vi "Control_PP_Blocks.vi"() -> (5 "Plug in titles":string[](array[string]), 7 "Plug in values":string[](array[string]))   [LabVIEW 2022 SP3]
uses:
  Globals/Meas_global.vi
  Post_Processing_specials/Block_Control_global.vi
panel:
  in  "No of Blocks to PP":i32=1 min=1
  in  "Start Block Number":i32=1 min=1
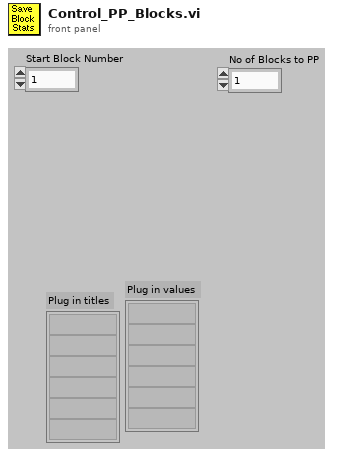
[diagram p1: front panel]
types:
  T1 = typedef "Post_Process.ctl" = enum16{"Take New Data", "Post Process Raw Data File"}
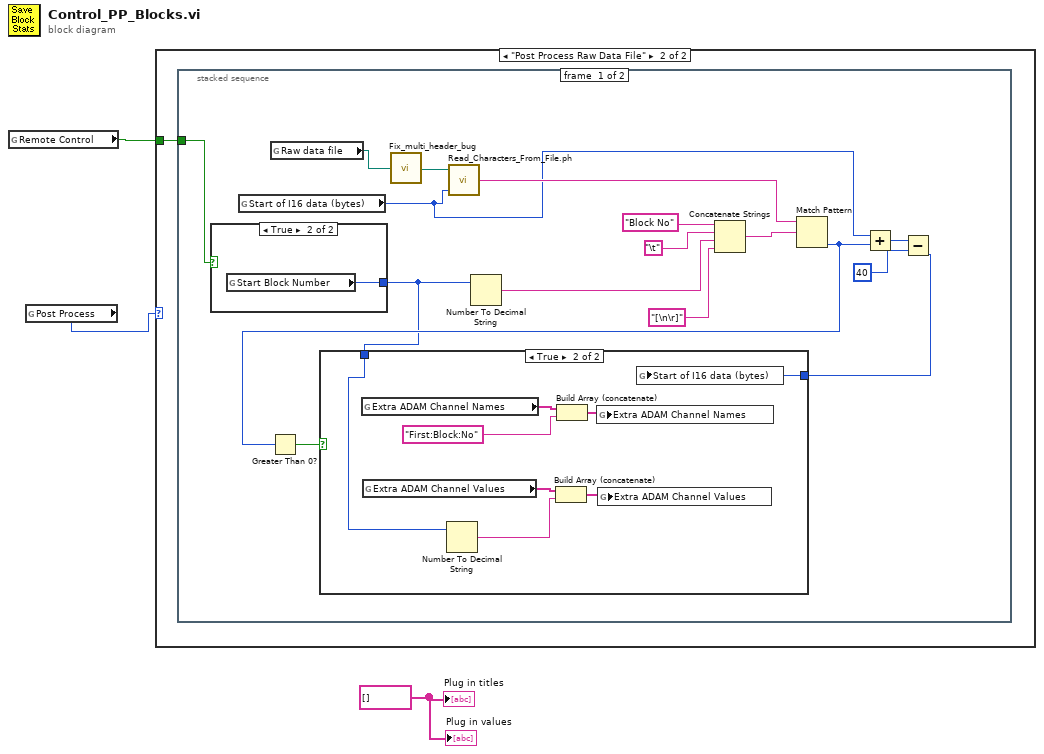
[diagram p0: block diagram]
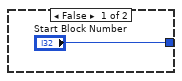
[diagram p3: hidden frame]
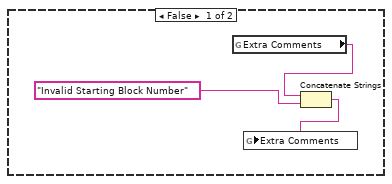
[diagram p4: hidden frame]
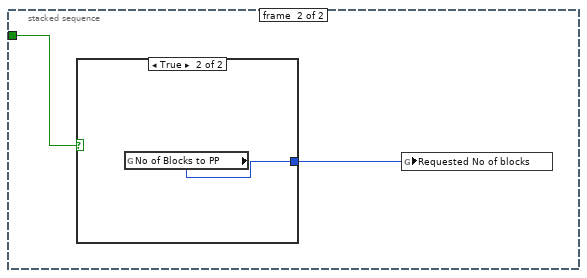
[diagram p5: hidden frame]
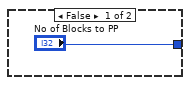
[diagram p6: hidden frame]
diagram:
  w2 = string[] [] ("Plug in titles")
  n1 = global read "Block_Control_global.vi" "Remote Control"() -> (w1:bool)
  n2 = global read "Meas_global.vi" "Post Process"() -> (w3:T1)
  n3 = case shown="\"Post Process Raw Data File\"" w3 {
    tunnel: w1 -> [_ w4]
    frame "Take New Data" {
    }
    frame "Post Process Raw Data File" {
      n4 = stacked-sequence {
        tunnel: w4 -> [w6 w34]
        frame #0 {
          n5 = case shown="True" w6 {
            tunnel: ["Start Block Number" w22] -> w5
            frame False {
            }
            frame True {
              n6 = global read "Block_Control_global.vi" "Start Block Number"() -> (w22:i32)
            }
          }
          n7 = global read "Meas_global.vi" "Start of I16 data (bytes)"() -> (w12:i64)
          n8 = global read "Meas_global.vi" "Raw data file"() -> (w20:path)
          n9 = call "Fix_multi_header_bug.vi"("Raw data File to Read"=w20) -> ("Raw data File to Read Out"=w19:path)
          n10 = call "Read_Characters_From_File.ph.vi"("file path (dialog if empty)"=w19, "start of read offset (chars.: 0)"=w12) -> ("character string"=w14:string)  [unwired: 4 in, 3 out]
          n11 = Number To Decimal String(number=w5) -> (decimal integer string=w16:string)  [unwired: 1 in]
          n12 = Concatenate Strings("Block No", "\t", w16, "[\n\r]") -> (w15:string)
          n13 = Match Pattern(string=w14, regular expression=w15) -> (offset past match=w9:i32)  [unwired: 1 in, 3 out]
          n14 = Greater Than 0?(x=w9) -> (x > 0?=w8:bool)
          n15 = Add(x=w12, y=w9) -> (x+y=w11:i64)
          n16 = Subtract(x=w11, y=40) -> (x-y=w7:i64)
          n17 = case shown="True" w8 {
            tunnel: w7 -> [_ w33]
            tunnel: w5 -> [_ w27]
            frame False {
              n18 = global read "Meas_global.vi" "Extra Comments"() -> (w24:string)
              n19 = Concatenate Strings(w24, "Invalid Starting Block Number") -> (w25:string)
              n20 = global write "Meas_global.vi" "Extra Comments"(w25) -> ()
            }
            frame True {
              n21 = global read "Meas_global.vi" "Extra ADAM Channel Names"() -> (w32:string[])
              n22 = global read "Meas_global.vi" "Extra ADAM Channel Values"() -> (w28:string[])
              n23 = Number To Decimal String(number=w27) -> (decimal integer string=w26:string)  [unwired: 1 in]
              n24 = Build Array (concatenate)(w28, w26) -> (w29:string[])
              n25 = Build Array (concatenate)(w32, "First:Block:No") -> (w30:string[])
              n26 = global write "Meas_global.vi" "Extra ADAM Channel Names"(w30) -> ()
              n27 = global write "Meas_global.vi" "Extra ADAM Channel Values"(w29) -> ()
              n28 = global write "Meas_global.vi" "Start of I16 data (bytes)"(w33) -> ()
            }
          }
        }
        frame #1 {
          n29 = case shown="True" w34 {
            tunnel: ["No of Blocks to PP" w37] -> w35
            frame False {
            }
            frame True {
              n30 = global read "Block_Control_global.vi" "No of Blocks to PP"() -> (w37:i32)
            }
          }
          n31 = global write "Meas_global.vi" "Requested No of blocks"(w35) -> ()
        }
      }
    }
  }
  "Plug in values" <- w2
  "Plug in titles" <- w2
